vi "Aync Communication.vi"(11 "Input Data":T1) -> ()   [LabVIEW 2015, in "Shared Variable Custom Device.lvlib"]
uses:
  Shared Variable Custom Device.lvlib
  Input Data Control.ctl
  <vilib>/Utility/VariantDataType/Type.ctl
  Shared Variable/Shared Variable Cluster.ctl
  <vilib>/NI Veristand/Custom Device Tools/Custom Device Utility Library/Custom Device Utility Library.lvlib
  <vilib>/Utility/VariantDataType/VariantType.lvlib
panel:
  out "error out":errorcluster
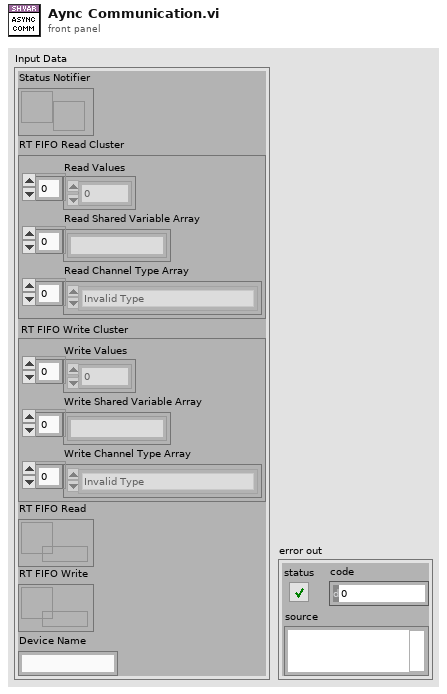
[diagram p1: front panel]
types:
  T1 = typedef "Shared Variable Custom Device.lvlib/Input Data Control.ctl" = cluster{"Status Notifier":refnum<notifier>, "RT FIFO Read Cluster":cluster{"Read Values":dbl[], "Read Shared Variable Array":string[], "Read Channel Type Array":T2[]}, "RT FIFO Write Cluster":cluster{"Write Values":dbl[], "Write Shared Variable Array":string[], "Write Channel Type Array":T2[]}, "RT FIFO Read":refnum<k33>, "RT FIFO Write":refnum<k33>, "Device Name":string}
  T2 = typedef "VariantType.lvlib/Type.ctl" = enum8{"Invalid Type", "Void", "I8", "I16", "I32", "I64", "U8", "U16", "U32", "U64", "Single Float", "Double Float", "Extended Float", "Single Complex", "Double Complex", "Extended Complex", "Enum U8", "Enum U16", "Enum U32", "Enum U64", "Single Float With Unit", "Double Float With Unit", "Extended Float With Unit", "Single Complex with Unit", "Double Complex with Unit", "Extended Complex with Unit", "Boolean", "String", "Path", "Picture", "Tag", "Array", "Cluster", "Variant", "LV Variant", "Waveform", "Timestamp", "Digital Waveform", "Digital Data", "ExpressData", "Refnum", "External Data", "VI", "Poly VI", "LabVIEW Class Instance", "Fixed Point"}
  T3 = cluster{"Read Access":enum8{"Allowed", "Required", "None"}, "Write Access":enum8{"Allowed", "Required", "None"}}
  T4 = typedef "Shared Variable Custom Device.lvlib/Shared Variable Cluster.ctl" = cluster{"Num Array":refnum<k21>[], "Num Array Index":i32[], "String Array":refnum<k21>[], "String Array Index":i32[], "Bool Array":refnum<k21>[], "Bool Array Index":i32[]}
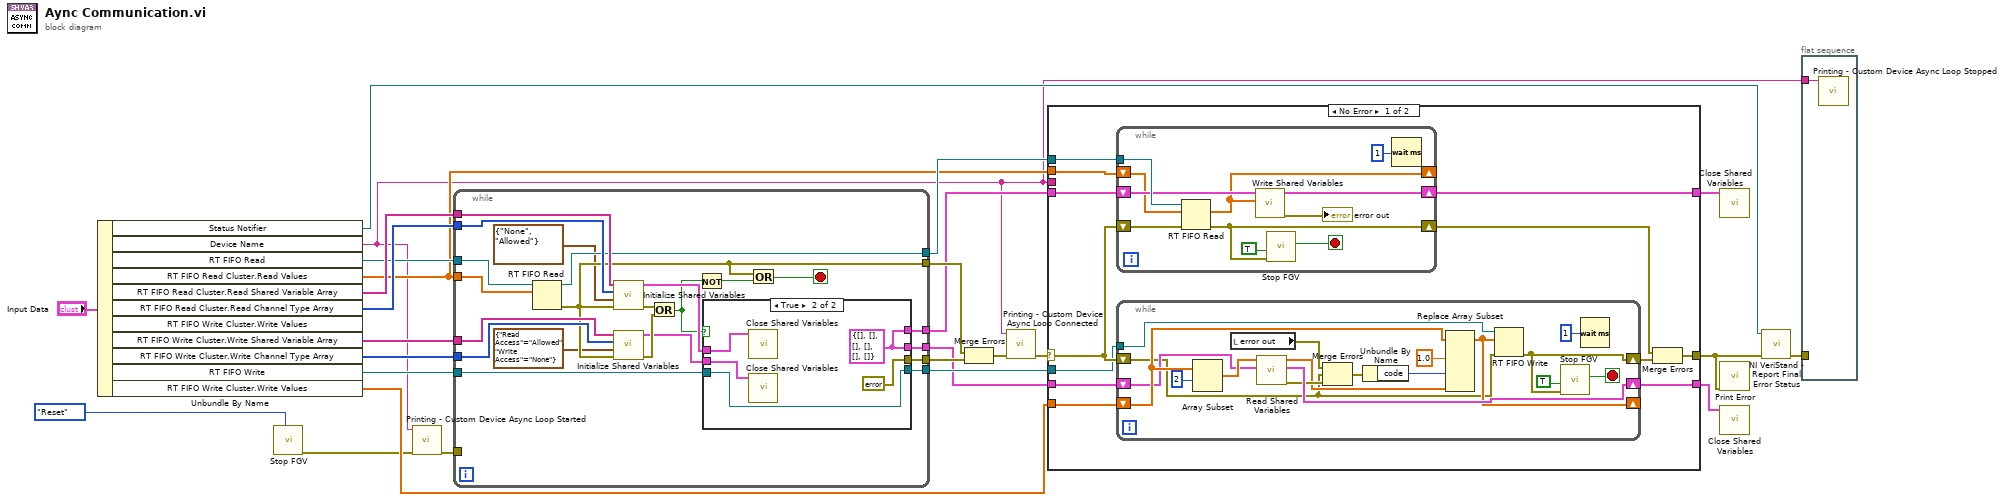
[diagram p0: block diagram]
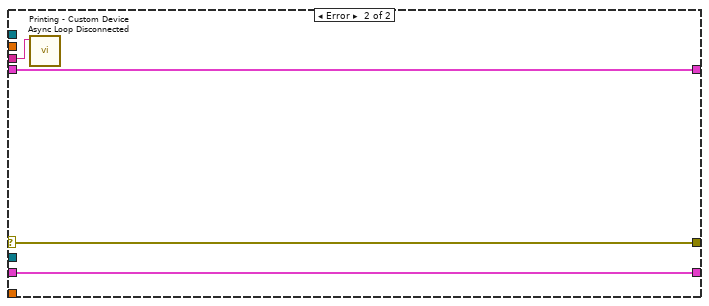
[diagram p2: hidden frame]
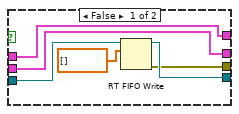
[diagram p3: hidden frame]
diagram:
  n1 = Unbundle By Name("Input Data") -> ("Status Notifier"=w4:refnum<notifier>, "Device Name"=w3:string, "RT FIFO Read"=w21:refnum<k33>, "RT FIFO Read Cluster.Read Values"=w9:dbl[], "RT FIFO Read Cluster.Read Shared Variable Array"=w25:string[], "RT FIFO Read Cluster.Read Channel Type Array"=w24:T2[], "RT FIFO Write Cluster.Write Shared Variable Array"=w23:string[], "RT FIFO Write Cluster.Write Channel Type Array"=w22:T2[], "RT FIFO Write"=w20:refnum<k33>, "RT FIFO Write Cluster.Write Values"=w5:dbl[])  [unwired: 1 out]
  n2 = call "Stop FGV.vi"("Command"=enum16{"Write", "Read", "Reset"}."Reset") -> ("error out"=w2:errorcluster)  [unwired: 8 in, 2 out]
  n3 = call "Printing - Custom Device Async Loop Started.vi"("error in (no error)"=w2, "Name"=w3) -> ("error out"=w8:errorcluster)  [unwired: 9 in]
  n4 = while {
    tunnel: w25 -> [w48]
    tunnel: w24 -> [w47]
    tunnel: w23 -> [w46]
    tunnel: w22 -> [w45]
    tunnel: [w39] -> w16
    tunnel: [w38] -> w13
    tunnel: w21 -> [w37]
    tunnel: w9 -> [w36]
    tunnel: w20 -> [w33]
    tunnel: [w32] -> w14
    tunnel: [w31] -> w17
    tunnel: [w30] -> w19
    tunnel: [w29] -> w18
    tunnel: w8 -> [_]
    stop <- w34 stop-if-true
    n5 = RT FIFO Read(0:w37, 1:w36) -> (8:w31:refnum<k33>, 11:w30:errorcluster)  [unwired: 2 in, 3 out]
    n6 = call "Initialize Shared Variables.vi"("error in (no error)"=w30, "Access"=T3 {"Read Access"=enum."None", "Write Access"=enum."Allowed"}, "Channel Type Array"=w47, "Shared Variable Array"=w48) -> ("error out"=w44:errorcluster, "Shared Variable Cluster"=w43:T4)  [unwired: 6 in]
    n7 = call "Initialize Shared Variables.vi"("error in (no error)"=w30, "Access"=T3 {"Read Access"=enum."Allowed", "Write Access"=enum."None"} ("access"), "Channel Type Array"=w45, "Shared Variable Array"=w46) -> ("error out"=w42:errorcluster, "Shared Variable Cluster"=w41:T4)  [unwired: 6 in]
    n8 = Or(x=w44, y=w42) -> (x .or. y?=w40:bool)
    n9 = Not(x=w40) -> (.not. x?=w35:bool)
    n10 = case shown="True" w40 {
      tunnel: w43 -> [w54 w59]
      tunnel: w41 -> [w53 w58]
      tunnel: [w54 w57] -> w39
      tunnel: [w53 w57] -> w38
      tunnel: w33 -> [w52 w56]
      tunnel: [w50 w56] -> w32
      tunnel: [w49 errorcluster {"status"=FALSE, "code"=0, "source"=""} ("error out")] -> w29
      frame False {
        n11 = RT FIFO Write(0:w52, 1:dbl[] [] ("element")) -> (8:w50:refnum<k33>, 11:w49:errorcluster)  [unwired: 3 in, 2 out]
      }
      frame True {
        w57 = T4 {"Num Array"=[], "Num Array Index"=[], "String Array"=[], "String Array Index"=[], "Bool Array"=[], "Bool Array Index"=[]} ("Shared Variable Cluster")
        n12 = call "Close Shared Variables.vi"("Shared Variable Cluster"=w59) -> ()  [unwired: 10 in, 1 out]
        n13 = call "Close Shared Variables.vi"("Shared Variable Cluster"=w58) -> ()  [unwired: 10 in, 1 out]
      }
    }
    n14 = Or(x=w30, y=w35) -> (x .or. y?=w34:bool)
  }
  n15 = Merge Errors(w19, w18) -> (w6:errorcluster)
  n16 = call "Printing - Custom Device Async Loop Connected.vi"("error in (no error)"=w6, "Name"=w3) -> ("error out"=w7:errorcluster)  [unwired: 9 in]
  n17 = case shown="No Error" w7 {
    selector: w7 -> [w67 w101]
    tunnel: w17 -> [w71 _]
    tunnel: w16 -> [w70 w104]
    tunnel: [w69 w104] -> w15
    tunnel: w5 -> [w68 _]
    tunnel: w14 -> [w66 _]
    tunnel: w13 -> [w65 w103]
    tunnel: [w64 w103] -> w12
    tunnel: [w61 w101] -> w10
    tunnel: w9 -> [w60 _]
    tunnel: w3 -> [_ w102]
    frame No Error {
      n18 = while {
        tunnel: w71 -> [w100]
        shift-right: [w91] -> w63
        shift-left: w67 -> [w99]
        shift-right: [w93] -> w69
        shift-left: w70 -> [w98]
        shift-right: [w92] -> _
        shift-left: w60 -> [w94]
        stop <- w96 stop-if-true
        n19 = RT FIFO Read(0:w100, 1:w94, 3:w99) -> (9:w92:dbl[], 11:w91:errorcluster)  [unwired: 1 in, 3 out]
        n20 = call "Write Shared Variables.vi"("Read Values"=w92, "Shared Variables to Write in"=w98) -> ("error out"=→"error out":errorcluster, "Shared Variables to Write out"=w93:T4)  [unwired: 8 in]
        n21 = call "Stop FGV.vi"("error in (no error)"=w91, "Stop on Error?"=TRUE) -> ("Latched Stop"=w96:bool)  [unwired: 7 in, 2 out]
        n22 = Wait (ms)(milliseconds to wait=u32 1) -> ()  [unwired: 1 out]
      }
      n23 = while {
        shift-right: [w78] -> _
        shift-left: w68 -> [w86]
        shift-right: [w73] -> w62
        shift-left: w67 -> [w74]
        tunnel: w66 -> [w85]
        shift-right: [w81] -> w64
        shift-left: w65 -> [w82]
        stop <- w83 stop-if-true
        n24 = Array Subset(array=w86, index=2) -> (w88:dbl[])  [unwired: 1 in]
        n25 = local read "error out"() -> (w80:errorcluster)
        n26 = call "Read Shared Variables.vi"("Shared Variables To Read in"=w82, "Write Values in"=w88) -> ("error out"=w79:errorcluster, "Shared Variables To Read out"=w81:T4, "Write Values out"=w75:dbl[])  [unwired: 7 in]
        n27 = Merge Errors(w80, w74, w79) -> (w77:errorcluster)
        n28 = Unbundle By Name(w77) -> ("code"=w76:i32)
        n29 = Replace Array Subset(array=w86, new element #1=1.0 ("t"), new element #2=w76, new element #3=w75) -> (w78:dbl[])  [unwired: 3 in]
        n30 = RT FIFO Write(0:w85, 1:w78, 3:w74) -> (11:w73:errorcluster)  [unwired: 2 in, 3 out]
        n31 = call "Stop FGV.vi"("error in (no error)"=w73, "Stop on Error?"=TRUE) -> ("Latched Stop"=w83:bool)  [unwired: 7 in, 2 out]
        n32 = Wait (ms)(milliseconds to wait=u32 1) -> ()  [unwired: 1 out]
      }
      n33 = Merge Errors(w63, w62) -> (w61:errorcluster)
    }
    frame Error {
      n34 = call "Printing - Custom Device Async Loop Disconnected.vi"("Name"=w102) -> ()  [unwired: 10 in, 1 out]
    }
  }
  n35 = call "Close Shared Variables.vi"("Shared Variable Cluster"=w15) -> ()  [unwired: 10 in, 1 out]
  n36 = call "Print Error.vi"("error in (no error)"=w10) -> ()  [unwired: 11 in]
  n37 = call "Close Shared Variables.vi"("Shared Variable Cluster"=w12) -> ()  [unwired: 10 in, 1 out]
  n38 = call <vilib>:"NI VeriStand - Report Final Error Status.vi"("error in (no error)"=w10, "Status Notifier"=w4) -> ("error out"=w11:errorcluster)  [unwired: 9 in]
  n39 = flat-sequence {
    tunnel: w11 -> [_]
    tunnel: w3 -> [w105]
    frame #0 {
      n40 = call "Printing - Custom Device Async Loop Stopped.vi"("Name"=w105) -> ()  [unwired: 10 in, 1 out]
    }
  }
